vi "FTW-TransferClient-DownloadBegin.vi"(0 "TransferClient.dotNET":refnum<class "FTW-TransferClient-dotNET.lvclass">, 5 "Local Filepath":path, 7 "Remote Relative Filepath":string, 11 "error in":errorcluster) -> (4 "TransferClient.dotNET out":refnum<class "FTW-TransferClient-dotNET.lvclass">, 6 "Download Events":refnum<event-registration>, 15 "error out":errorcluster)   [LabVIEW 2015, in "FTW-TransferClient-dotNET.lvclass"]
uses:
  FTW-TransferClient-dotNET.lvclass
  FTW-TransferClient-TransferProgress.ctl
  FTW-TransferClient-TransferStatus.ctl
  FTW-TransferClient-dotNET.lvclass/FTW-TransferClient-dotNET.ctl
  FTW-TransferClient.lvclass
panel:
  # "Inputs"
  # "Outputs"
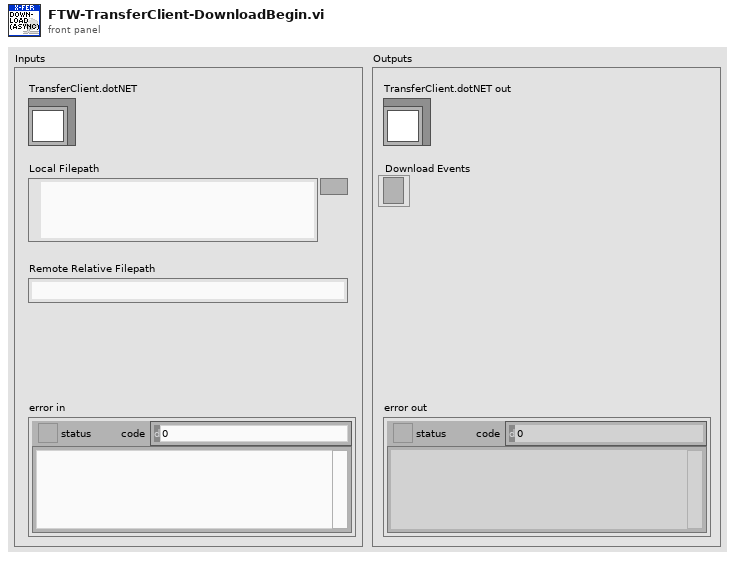
[diagram p1: front panel]
types:
  T1 = cluster{"Transfer Progress":refnum<user-event>, "Transfer Begin Timestamp":u32, "AbsoluteURI":string, "Local Filepath":path}
  T2 = cluster{"Transfer Complete":refnum<user-event>, "Transfer Begin Timestamp":u32, "AbsoluteURI":string, "Local Filepath":path}
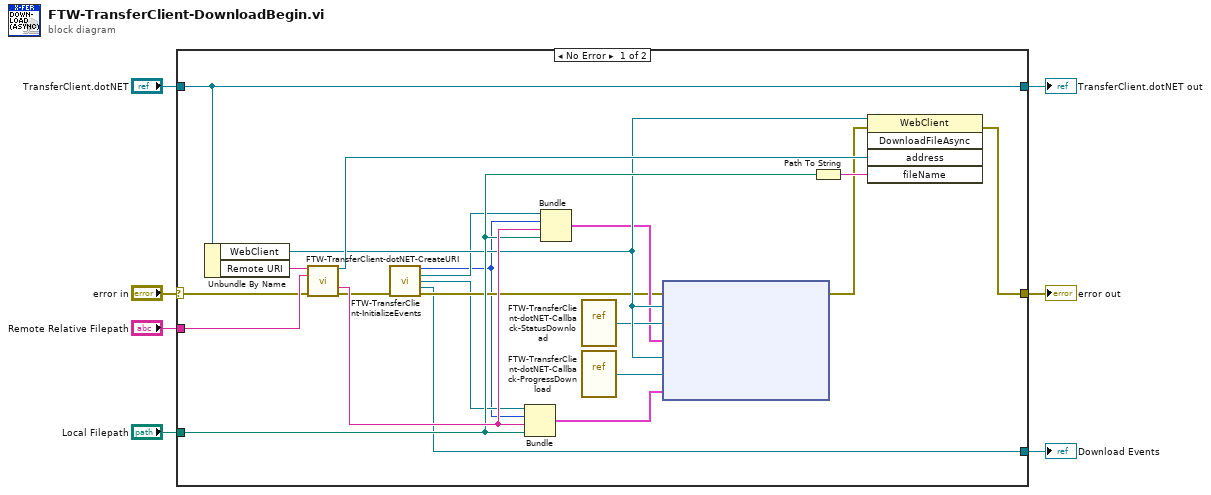
[diagram p0: block diagram]
diagram:
  n1 = case shown="No Error" "error in" {
    selector: "error in" -> [w21 w29]
    tunnel: "TransferClient.dotNET" -> [w24 w30]
    tunnel: [w18 w29] -> w7
    tunnel: [w24 w30] -> w6
    tunnel: "Remote Relative Filepath" -> [w23 _]
    tunnel: "Local Filepath" -> [w22 _]
    tunnel: [w8 _] -> w1
    frame No Error {
      n2 = Unbundle By Name(w24) -> ("WebClient"=w17:refnum<k24>, "Remote URI"=w27:string)
      n3 = call "FTW-TransferClient-dotNET-CreateURI.vi"("URI"=w27, "Relative URI"=w23, "error in"=w21) -> ("URI ref"=w26:refnum<k24>, "AbsoluteURI"=w25:string, "error out"=w13:errorcluster)  [unwired: 7 in, 3 out]
      n4 = call "FTW-TransferClient-InitializeEvents.vi"("error in"=w13) -> ("Transfer Begin Timestamp"=w9:u32, "Transfer Complete"=w11:refnum<user-event>, "Transfer Progress"=w10:refnum<user-event>, "Transfer Events"=w8:refnum<event-registration>, "error out"=w12:errorcluster)  [unwired: 10 in]
      n5 = Bundle("Transfer Progress"=w10, "Transfer Begin Timestamp"=w9, "AbsoluteURI"=w25, "Local Filepath"=w22) -> (w20:T1)  [unwired: 1 in]
      n6 = Bundle("Transfer Complete"=w11, "Transfer Begin Timestamp"=w9, "AbsoluteURI"=w25, "Local Filepath"=w22) -> (w14:T2)  [unwired: 1 in]
      n7 = vi-ref "FTW-TransferClient-dotNET-Callback-StatusDownload.vi"() -> ("vi reference"=w15:refnum<vi>)
      n8 = vi-ref "FTW-TransferClient-dotNET-Callback-ProgressDownload.vi"() -> ("vi reference"=w16:refnum<vi>)
      n9 = node(w12, w17, w15, w14, w17, w16, w20) -> (w19:errorcluster)  [unwired: 1 in, 1 out]
      n10 = Path To String(path=w22) -> (string=w28:string)
      n11 = invoke class="WebClient" method="DownloadFileAsync"(reference=w17, error in=w19, "address"=w26, "fileName"=w28) -> (error out=w18:errorcluster)  [unwired: 1 in, 4 out]
    }
    frame Error {
    }
  }
  "error out" <- w7
  "TransferClient.dotNET out" <- w6
  "Download Events" <- w1
